vi "IR_LearnEventCreate.vi"(8 "error in (no error)":errorcluster, 11 "Devices In":u64[](array[numeric])) -> (0 "error out":errorcluster, 2 "Event Registration Refnum":refnum<event-registration>, 3 "Devices Out":u64[](array[numeric]))   [LabVIEW 2012, in "Phidget IR.lvlib"]
doc: "${Learn:CreateHeader}"
uses:
  <instrlib>/Phidgets/Phidget IR/Phidget IR.lvlib
  <instrlib>/Phidgets/Phidget IR/Public/CodeInfo.ctl
  <instrlib>/Phidgets/Phidget Common/Phidget Common.lvlib
  phidget22.dll
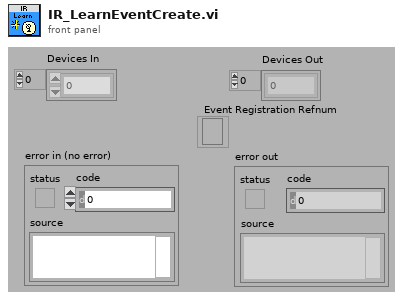
[diagram p1: front panel]
types:
  T1 = typedef "Phidget IR.lvlib/CodeInfo.ctl" = cluster{"bitCount":u32, "encoding":u32, "length":u32, "gap":u32, "trail":u32, "header[0]":u32, "header[1]":u32, "one[0]":u32, "one[1]":u32, "zero[0]":u32, "zero[1]":u32, "repeat[0]":u32, "repeat[1]":u32, "repeat[2]":u32, "repeat[3]":u32, "repeat[4]":u32, "repeat[5]":u32, "repeat[6]":u32, "repeat[7]":u32, "repeat[8]":u32, "repeat[9]":u32, "repeat[10]":u32, "repeat[11]":u32, "repeat[12]":u32, "repeat[13]":u32, "repeat[14]":u32, "repeat[15]":u32, "repeat[16]":u32, "repeat[17]":u32, "repeat[18]":u32, "repeat[19]":u32, "repeat[20]":u32, "repeat[21]":u32, "repeat[22]":u32, "repeat[23]":u32, "repeat[24]":u32, "repeat[25]":u32, "minRepeat":u32, "dutyCycle":dbl, "carrierFrequency":u32, "toggleMask[0]":i8, "toggleMask[1]":i8, "toggleMask[2]":i8, "toggleMask[3]":i8, "toggleMask[4]":i8, "toggleMask[5]":i8, "toggleMask[6]":i8, "toggleMask[7]":i8, "toggleMask[8]":i8, "toggleMask[9]":i8, "toggleMask[10]":i8, "toggleMask[11]":i8, "toggleMask[12]":i8, "toggleMask[13]":i8, "toggleMask[14]":i8, "toggleMask[15]":i8, "toggleMask[16]":i8, "toggleMask[17]":i8, "toggleMask[18]":i8, "toggleMask[19]":i8, "toggleMask[20]":i8, "toggleMask[21]":i8, "toggleMask[22]":i8, "toggleMask[23]":i8, "toggleMask[24]":i8, "toggleMask[25]":i8, "toggleMask[26]":i8, "toggleMask[27]":i8, "toggleMask[28]":i8, "toggleMask[29]":i8, "toggleMask[30]":i8, "toggleMask[31]":i8, "toggleMask[32]":i8}
  T2 = cluster{"phid":u64, "codeStr":string, "codeInfo":T1}
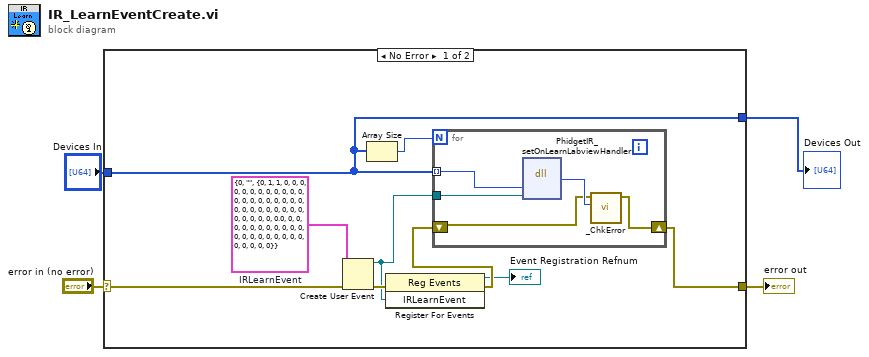
[diagram p0: block diagram]
diagram:
  n1 = case shown="No Error" "error in (no error)" {
    selector: "error in (no error)" -> [w13 w20]
    tunnel: [w9 w20] -> w3
    tunnel: "Devices In" -> [w11 w19]
    tunnel: [w11 w19] -> w1
    frame No Error {
      w7 = T2 {"phid"=0, "codeStr"="", "codeInfo"={"bitCount"=0, "encoding"=1, "length"=1, "gap"=0, "trail"=0, "header[0]"=0, "header[1]"=0, "one[0]"=0, "one[1]"=0, "zero[0]"=0, "zero[1]"=0, "repeat[0]"=0, "repeat[1]"=0, "repeat[2]"=0, "repeat[3]"=0, "repeat[4]"=0, "repeat[5]"=0, "repeat[6]"=0, "repeat[7]"=0, "repeat[8]"=0, "repeat[9]"=0, "repeat[10]"=0, "repeat[11]"=0, "repeat[12]"=0, "repeat[13]"=0, "repeat[14]"=0, "repeat[15]"=0, "repeat[16]"=0, "repeat[17]"=0, "repeat[18]"=0, "repeat[19]"=0, "repeat[20]"=0, "repeat[21]"=0, "repeat[22]"=0, "repeat[23]"=0, "repeat[24]"=0, "repeat[25]"=0, "minRepeat"=0, "dutyCycle"=0.0, "carrierFrequency"=0, "toggleMask[0]"=0, "toggleMask[1]"=0, "toggleMask[2]"=0, "toggleMask[3]"=0, "toggleMask[4]"=0, "toggleMask[5]"=0, "toggleMask[6]"=0, "toggleMask[7]"=0, "toggleMask[8]"=0, "toggleMask[9]"=0, "toggleMask[10]"=0, "toggleMask[11]"=0, "toggleMask[12]"=0, "toggleMask[13]"=0, "toggleMask[14]"=0, "toggleMask[15]"=0, "toggleMask[16]"=0, "toggleMask[17]"=0, "toggleMask[18]"=0, "toggleMask[19]"=0, "toggleMask[20]"=0, "toggleMask[21]"=0, "toggleMask[22]"=0, "toggleMask[23]"=0, "toggleMask[24]"=0, "toggleMask[25]"=0, "toggleMask[26]"=0, "toggleMask[27]"=0, "toggleMask[28]"=0, "toggleMask[29]"=0, "toggleMask[30]"=0, "toggleMask[31]"=0, "toggleMask[32]"=0}}  # IRLearnEvent
      n2 = Create User Event(user event datatype=w7, error in=w13) -> (user event=w6:refnum<user-event>, error out=w12:errorcluster)
      n3 = Array Size(array=w11) -> (size(s)=w8:i32)
      n4 = register-events(error in=w12, w6) -> (reference out=→"Event Registration Refnum":refnum<event-registration>, error out=w10:errorcluster)  [unwired: 1 in]
      n5 = for {
        N: w8 -> [_]
        tunnel: w11 -> [w16] mode=indexing
        shift-right: [w18] -> w9
        shift-left: w10 -> [w15]
        tunnel: w6 -> [w14]
        n6 = dll-call lib="phidget22.*" fn="PhidgetIR_setOnLearnLabviewHandler"("phid"=w16, "AcceEvent"=w14) -> ("return type"=w17:i32)  [unwired: 5 in, 2 out]
        n7 = call <instrlib>:"_ChkError.vi"("Return Code"=w17, "error in (no error)"=w15) -> ("error out"=w18:errorcluster)  [unwired: 9 in]
      }
    }
    frame Error {
    }
  }
  "error out" <- w3
  "Devices Out" <- w1
